vi "Do.vi"(8 "error in (no error)":errorcluster, 10 "Actor in":refnum<class "Actor.lvclass">, 11 "SwitchOption Msg":refnum<class "SwitchOption Msg.lvclass">) -> (0 "error out":errorcluster, 2 "Actor out":refnum<class "Actor.lvclass">)   [LabVIEW 2015, in "Admin_Actor.lvlib" / "SwitchOption Msg.lvclass"]
doc: "This VI delivers the message to the actor by calling the appropriate method(s) on the actor."
uses:
  SwitchOption Msg.lvclass
  <vilib>/ActorFramework/Actor/Actor.lvclass
  Admin_Actor/Admin_Actor.lvclass
  User_Actor/Member_Actor Messages/SwitchOption Msg/SwitchOption Msg.lvclass/SwitchOption Msg.ctl
  User_Actor/Member_Actor Messages/SwitchOption Msg/SwitchOption Msg.lvclass
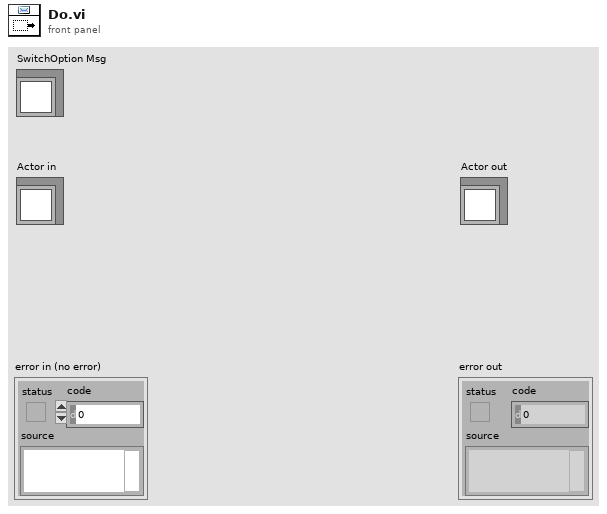
[diagram p1: front panel]
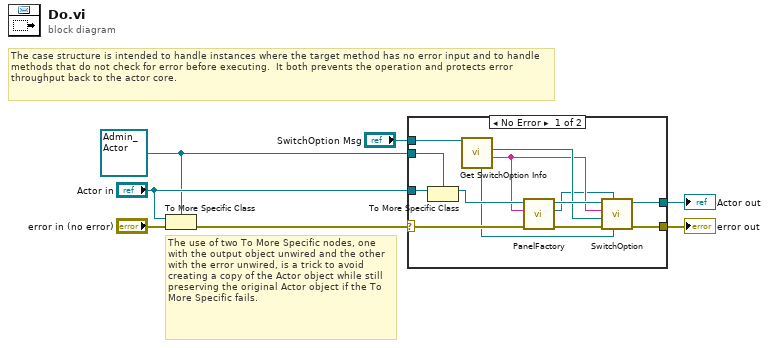
[diagram p0: block diagram]
diagram:
  w2 = refnum<class "Admin_Actor.lvclass"> refnum ("Actor in")
  # "The use of two To More Specific nodes, one with the output object unwired and the other with the error unwired, is a trick to avoid creating a copy of the Actor object while still preserving the original Actor object if the To More Specific fails."
  # "The case structure is intended to handle instances where the target method has no error input and to handle methods that do not check for error before executing.  It both prevents the operation and protects error throughput back to the actor core."
  n1 = To More Specific Class(target class=w2, reference="Actor in", error in="error in (no error)") -> (error out=w6:errorcluster)  [unwired: 1 out]
  n2 = case shown="No Error" w6 {
    selector: w6 -> [w15 w22]
    tunnel: [w20 w22] -> w5
    tunnel: [w19 w21] -> w4
    tunnel: "Actor in" -> [w18 w21]
    tunnel: w2 -> [w17 _]
    tunnel: "SwitchOption Msg" -> [w12 _]
    frame No Error {
      n3 = To More Specific Class(target class=w17, reference=w18) -> (specific class reference=w16:refnum<class "Admin_Actor.lvclass">)  [unwired: 1 in, 1 out]
      n4 = call "Get SwitchOption Info.vi"("SwitchOption Msg in"=w12) -> ("ThreadName(\"\")"=w9:string, "Base Path"=w11:path, "SubPanelRef"=w10:refnum<vi>)  [unwired: 6 in, 2 out]
      n5 = call-dynamic "PanelFactory.vi"("error in (no error)"=w15, "ThreadName(\"\")"=w9, "Admin_Actor in"=w16) -> ("error out"=w14:errorcluster, "MemberPanel(Product)"=w8:refnum<class "MemberPanel.lvclass">, "Admin_Actor out"=w13:refnum<class "Admin_Actor.lvclass">)  [unwired: 6 in]
      n6 = call-dynamic "SwitchOption.vi"("SubPanelRef"=w10, "Panel Controller"=w8, "error in (no error)"=w14, "Base Path"=w11, "ThreadName(\"\")"=w9, "Admin_Actor in"=w13) -> ("error out"=w20:errorcluster, "Admin_Actor out"=w19:refnum<class "Admin_Actor.lvclass">)  [unwired: 4 in]
    }
    frame Error {
      # "If type check fails, pass the original object out again."
    }
  }
  "error out" <- w5
  "Actor out" <- w4
